vi "SEK2020v1VI7IrAteRespectivaCor.vi"(3 "NXT/EV3 2":T2, 8 "Parâmetros 2":T1={"Azul Max EV3 Cor"=17, "Azul Min EV3 Cor"=0, "Verde Max EV3 Cor"=6, "Verde Min EV3 Cor"=0, "Vermelho Max Ev3 Cor"=0, "Vermelho Min EV3 Cor"=0, "Chão EV3 Cor"=0.0, "Branco Max EV3 Cor"=0.0, "Branco Min EV3 Cor"=0.0, "Preto Max EV3 Cor"=0.0, "Preto Min EV3 Cor"=0.0, "Distância Tubulação"=0.0, "Distância Frontal"=0.0, "Amarelo Max EV3 Cor"=0.0, "Amarelo Min EV3 Cor"=0.0, "Distância Lateral"=0.0, "90°"=0.0, "180°"=0.0, "Seguidor de Linha"=0.0}, 9 "Tam Tubo":i32) -> (11 "NXT/EV3":T2)   [LabVIEW 2016]
uses:
  <vilib>/NXT/Subs/LVHSConnector.ctl
  <vilib>/NXT/LegoClasses/BrickReference/BrickReference.lvclass
  <vilib>/NXT/Block Support/NXT_InputPort.ctl
  <vilib>/NXT/Dual Mode Library/Sensors/EV3_Color_Reflect.vi
  <vilib>/NXT/NXTIO Xnodes/AddressXNode/NXTIOAddress.xnode
panel:
  # "Sensor EV3 Cor"
  # "Sensor Ultrassônico"
  # "Sensor Giroscópio"
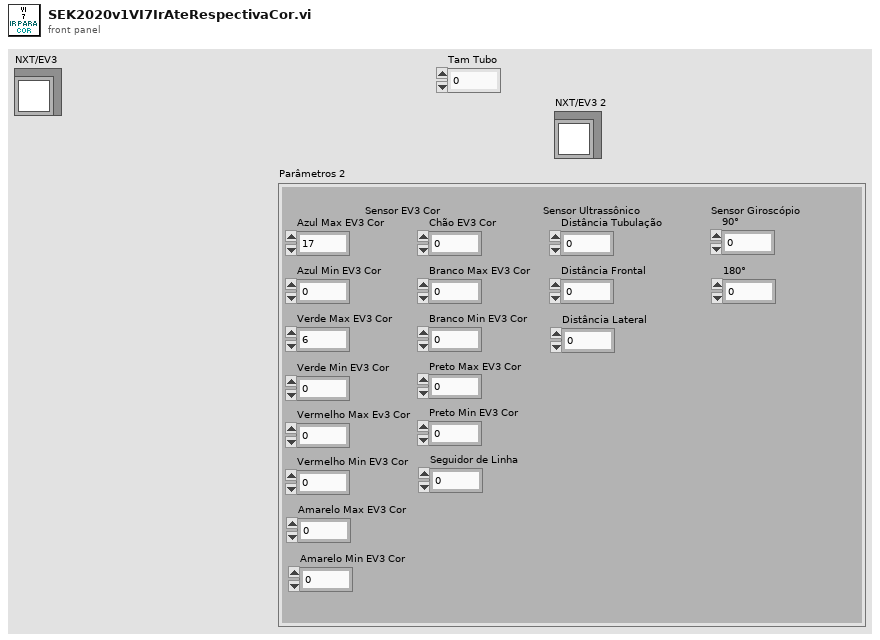
[diagram p1: front panel]
types:
  T1 = cluster{"Azul Max EV3 Cor":i32, "Azul Min EV3 Cor":i32, "Verde Max EV3 Cor":i32, "Verde Min EV3 Cor":i32, "Vermelho Max Ev3 Cor":i32, "Vermelho Min EV3 Cor":i32, "Chão EV3 Cor":sgl, "Branco Max EV3 Cor":sgl, "Branco Min EV3 Cor":sgl, "Preto Max EV3 Cor":sgl, "Preto Min EV3 Cor":sgl, "Distância Tubulação":sgl, "Distância Frontal":sgl, "Amarelo Max EV3 Cor":dbl, "Amarelo Min EV3 Cor":dbl, "Distância Lateral":sgl, "90°":sgl, "180°":sgl, "Seguidor de Linha":dbl}
  T2 = typedef "LVHSConnector.ctl" = refnum<class "BrickReference.lvclass">
  T3 = typedef "NXT_InputPort.ctl" = u32
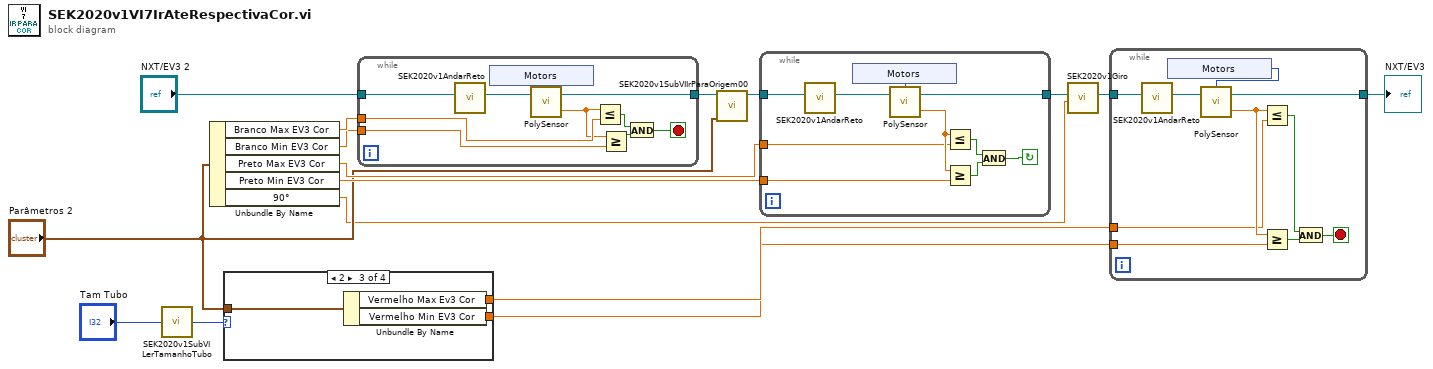
[diagram p0: block diagram]
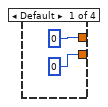
[diagram p2: hidden frame]
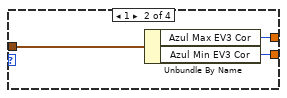
[diagram p3: hidden frame]
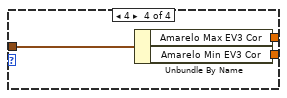
[diagram p4: hidden frame]
diagram:
  n1 = call "SEK2020v1SubVILerTamanhoTubo.vi"("TamTubo"="Tam Tubo") -> ("Numeric"=w6:i32)
  n2 = Unbundle By Name("Parâmetros 2") -> ("Branco Max EV3 Cor"=w16:sgl, "Branco Min EV3 Cor"=w15:sgl, "Preto Max EV3 Cor"=w14:sgl, "Preto Min EV3 Cor"=w13:sgl, "90°"=w1:sgl)
  n3 = case shown="2" w6 {
    tunnel: "Parâmetros 2" -> [_ w21 w24 w27]
    tunnel: [0 w20 w23 w26] -> w5
    tunnel: [0 w19 w22 w25] -> w4
    frame Default {
    }
    frame 1 {
      n4 = Unbundle By Name(w21) -> ("Azul Max EV3 Cor"=w20:i32, "Azul Min EV3 Cor"=w19:i32)
    }
    frame 2 {
      n5 = Unbundle By Name(w24) -> ("Vermelho Max Ev3 Cor"=w23:i32, "Vermelho Min EV3 Cor"=w22:i32)
    }
    frame 4 {
      n6 = Unbundle By Name(w27) -> ("Amarelo Max EV3 Cor"=w26:dbl, "Amarelo Min EV3 Cor"=w25:dbl)
    }
  }
  n7 = while {
    tunnel: "NXT/EV3 2" -> [w37]
    tunnel: w16 -> [w36]
    tunnel: w15 -> [w34]
    tunnel: [w29] -> w11
    stop <- w30 stop-if-true
    n8 = call "SEK2020v1AndarReto.vi"("NXT/EV3"=w37) -> ("NXT/EV3 2"=w33:T2)  [unwired: 9 in]
    n9 = xnode "Motors"() -> ("Sensor"=w28:T3)
    n10 = call-poly <vilib>:"PolySensor.vi"("NXT/EV3"=w33, "Port (Port 1)"=w28) -> ("Scaled Value"=w35:sgl, "NXT/EV3"=w29:T2)  [unwired: 1 in]
    n11 = Less Or Equal?(x=w35, y=w36) -> (x <= y?=w32:bool)
    n12 = Greater Or Equal?(x=w35, y=w34) -> (x >= y?=w31:bool)
    n13 = And(x=w32, y=w31) -> (x .and. y?=w30:bool)
  }
  n14 = call "SEK2020v1SubVIIrParaOrigem00.vi"("Parâmetros"="Parâmetros 2", "NXT/EV3"=w11) -> ("NXT/EV3 2"=w12:T2)  [unwired: 9 in]
  n15 = while {
    tunnel: w14 -> [w45]
    tunnel: w13 -> [w44]
    tunnel: w12 -> [w40]
    tunnel: [w42] -> w10
    stop <- w43 continue-if-true
    n16 = call "SEK2020v1AndarReto.vi"("NXT/EV3"=w40) -> ("NXT/EV3 2"=w39:T2)  [unwired: 9 in]
    n17 = xnode "Motors"() -> ("Sensor"=w41:T3)
    n18 = call-poly <vilib>:"PolySensor.vi"("NXT/EV3"=w39, "Port (Port 1)"=w41) -> ("Scaled Value"=w48:sgl, "NXT/EV3"=w42:T2)  [unwired: 1 in]
    n19 = Less Or Equal?(x=w48, y=w45) -> (x <= y?=w47:bool)
    n20 = Greater Or Equal?(x=w48, y=w44) -> (x >= y?=w46:bool)
    n21 = And(x=w47, y=w46) -> (x .and. y?=w43:bool)
  }
  n22 = call "SEK2020v1Giro.vi"("ANGULO"=w1, "NXT/EV3"=w10) -> ("NXT/EV3 2"=w9:T2)  [unwired: 6 in]
  n23 = while {
    tunnel: w9 -> [w57]
    tunnel: [w54] -> w8
    tunnel: w5 -> [w52]
    tunnel: w4 -> [w51]
    stop <- w55 stop-if-true
    n24 = call "SEK2020v1AndarReto.vi"("NXT/EV3"=w57) -> ("NXT/EV3 2"=w53:T2)  [unwired: 9 in]
    n25 = xnode "Motors"() -> ("Sensor"=w50:T3)
    n26 = call-poly <vilib>:"PolySensor.vi"("NXT/EV3"=w53, "Port (Port 1)"=w50) -> ("Scaled Value"=w58:sgl, "NXT/EV3"=w54:T2)  [unwired: 1 in]
    n27 = Less Or Equal?(x=w58, y=w52) -> (x <= y?=w59:bool)
    n28 = Greater Or Equal?(x=w58, y=w51) -> (x >= y?=w56:bool)
    n29 = And(x=w59, y=w56) -> (x .and. y?=w55:bool)
  }
  "NXT/EV3" <- w8
